vi "Extract IRF (Toeplitz).vi"(4 "balance parameter":dbl=5.0, 6 "Tail Smoothing (T)":bool=TRUE, 7 "Smoothing Order":i32=1, 8 "Error In":errorcluster, 9 "Time Constant":dbl, 10 "Intensity Array":dbl[](array[numeric]), 11 "t Array":dbl[](array[numeric])) -> (0 "Error Out":errorcluster, 1 "Message":string, 2 "IRF Array":dbl[](array[numeric]), 3 "t Array (dup)":dbl[](array[numeric]))   [LabVIEW 2021, in "Fits.lvlib"]
doc: "Extract IRF from provided decay and time constant"
uses:
  Fits.lvlib
  <vilib>/Analysis/baseanly.llb/Matrix Type of Inverse Matrix.ctl
  <vilib>/Analysis/baseanly.llb/A x Vector.vi
  <vilib>/Analysis/7linalg.llb/Create Special Real Matrix.vi
  <vilib>/Analysis/baseanly.llb/Real Inverse Matrix.vi
  <vilib>/Analysis/NI_AALPro.lvlib
  <vilib>/Analysis/NI_AALBase.lvlib
  <vilib>/ErrorRing/Error Ring.xnode
  <vilib>/Utility/error.llb/Error Cluster From Error Code.vi
  Graphs/XY Graph/XY Graph Add-Ons.lvlib
  Math/Math.lvlib
panel:
  out "Tail Min":dbl
  out "Tail Sum":dbl
  out "XY Graph":cluster{"t Array":dbl[], "Array":dbl[]}[](graph)
  # "see the AlliGator License on the block diagram (Ctrl+E or Window:Show Block Diagram)"
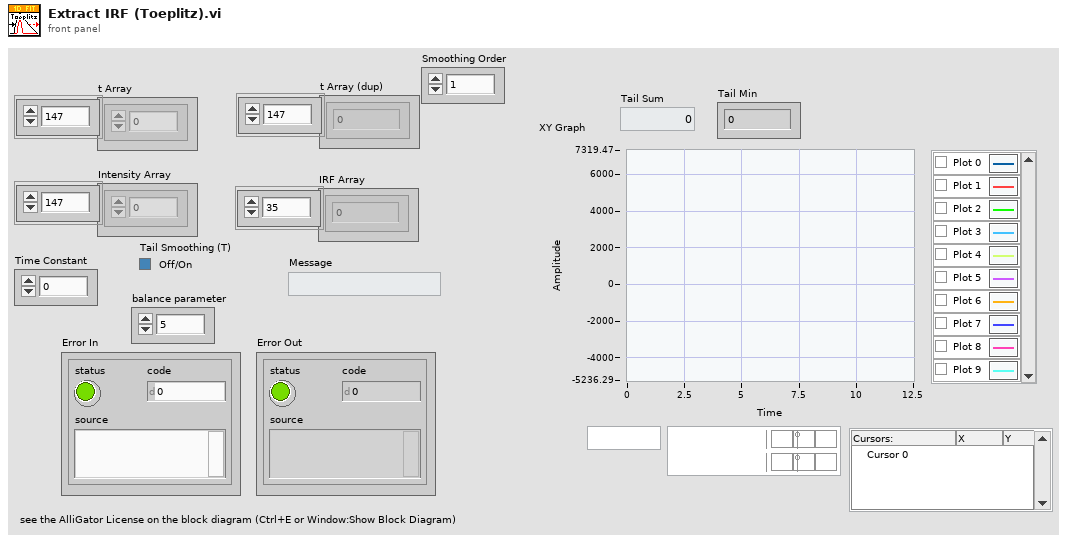
[diagram p1: front panel]
types:
  T1 = typedef "NI_AALBase.lvlib/Matrix Type of Inverse Matrix.ctl" = enum32{"General", "Positive Definite", "Lower Triangular", "Upper Triangular"}
  T2 = enum16{"Positive", "Positive w Noise", "Balanced"}
  T3 = typedef "NI_Matrix.lvlib/RealMatrix.ctl" = dbl[][]
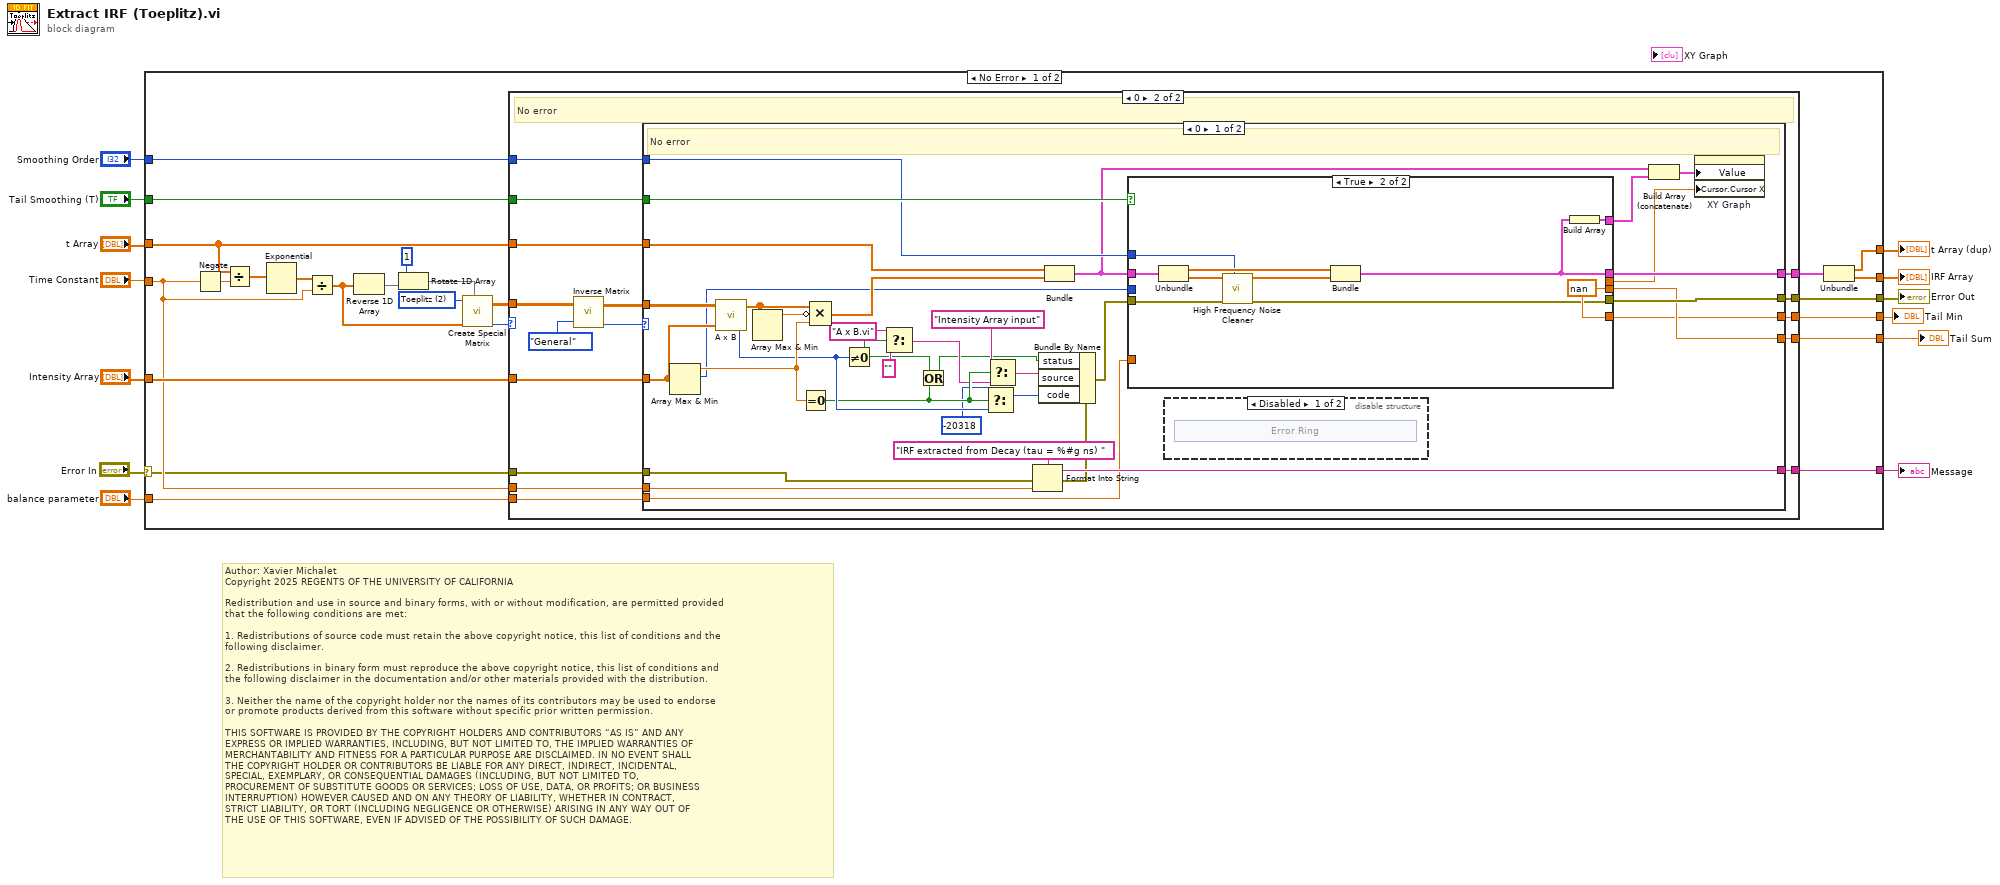
[diagram p0: block diagram]
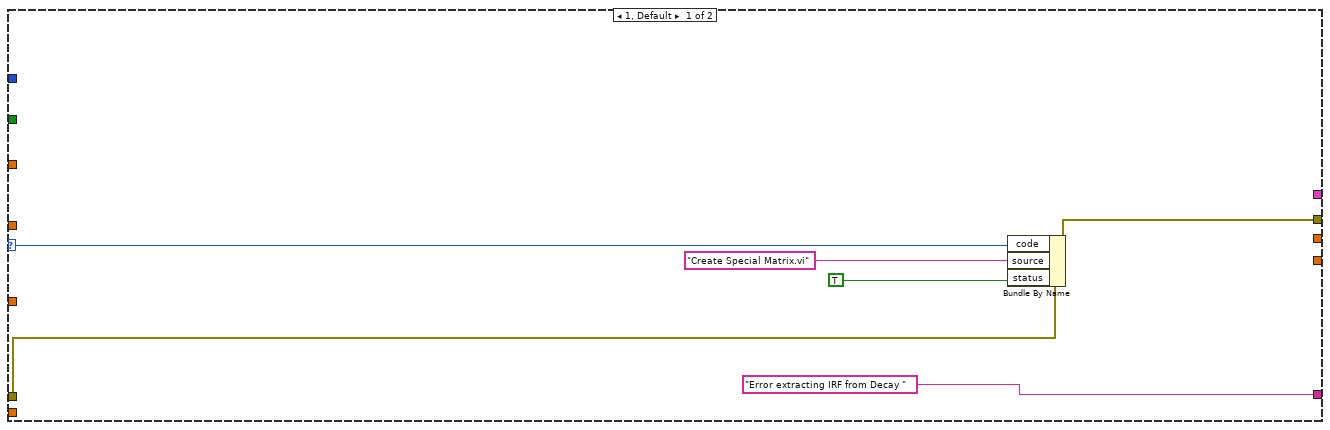
[diagram p2: hidden frame]
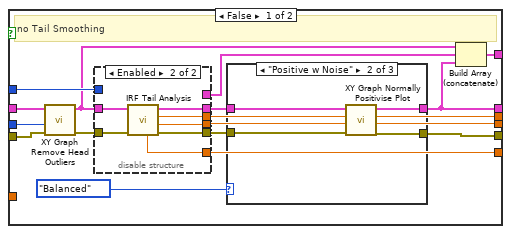
[diagram p4: hidden frame]
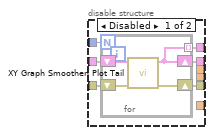
[diagram p5: hidden frame]
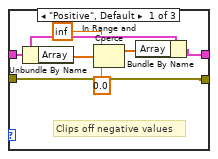
[diagram p6: hidden frame]
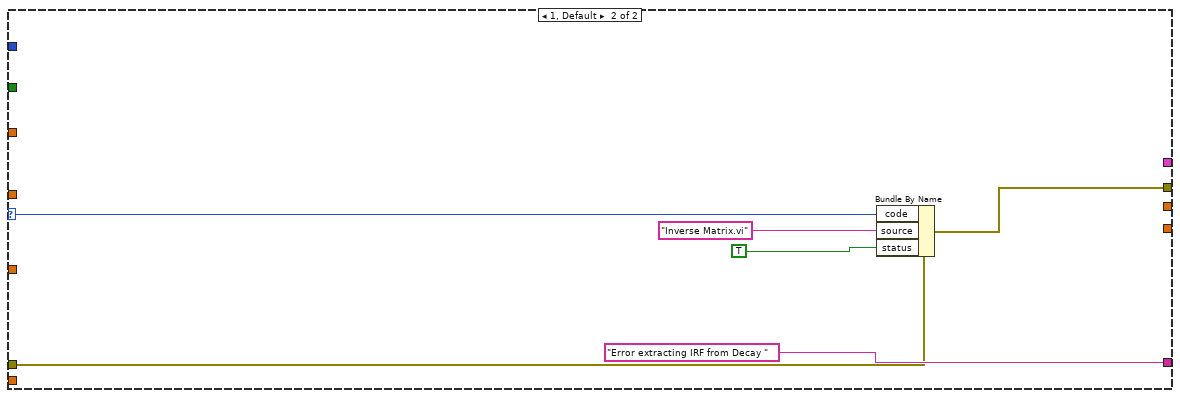
[diagram p8: hidden frame]
diagram:
  # "Author: Xavier Michalet\nCopyright 2025 REGENTS OF THE UNIVERSITY OF CALIFORNIA\n\nRedistribution and use in source and binary forms, with or without modification, are permitted provided\nthat the following conditions are met:\n\n1. Redistributions of source code must retain the above copyright notice, this list of conditions and the\nfollowing disclaimer.\n\n2. Redistributions in binary form must reproduce the above copyright notice, this list of conditions and\nthe following disclaimer in the documentation and/or other materials provided with the distribution.\n\n3. Neither the name of the copyright holder nor the names of its contributors may be used to endorse \nor promote products derived from this software without specific prior written permission.\n\nTHIS SOFTWARE IS PROVIDED BY THE COPYRIGHT HOLDERS AND CONTRIBUTORS “AS IS” AND ANY \nEXPRESS OR IMPLIED WARRANTIES, INCLUDING, BUT NOT LIMITED TO, THE IMPLIED WARRANTIES OF\nMERCHANTABILITY AND FITNESS FOR A PARTICULAR PURPOSE ARE DISCLAIMED. IN NO EVENT SHALL\nTHE COPYRIGHT HOLDER OR CONTRIBUTORS BE LIABLE FOR ANY DIRECT, INDIRECT, INCIDENTAL, \nSPECIAL, EXEMPLARY, OR CONSEQUENTIAL DAMAGES (INCLUDING, BUT NOT LIMITED TO, \nPROCUREMENT OF SUBSTITUTE GOODS OR SERVICES; LOSS OF USE, DATA, OR PROFITS; OR BUSINESS\nINTERRUPTION) HOWEVER CAUSED AND ON ANY THEORY OF LIABILITY, WHETHER IN CONTRACT, \nSTRICT LIABILITY, OR TORT (INCLUDING NEGLIGENCE OR OTHERWISE) ARISING IN ANY WAY OUT OF\nTHE USE OF THIS SOFTWARE, EVEN IF ADVISED OF THE POSSIBILITY OF SUCH DAMAGE."
  n1 = case shown="No Error" "Error In" {
    selector: "Error In" -> [w25 w162]
    tunnel: "Intensity Array" -> [w37 _]
    tunnel: "Time Constant" -> [w29 _]
    tunnel: "t Array" -> [w27 _]
    tunnel: [w24 w162] -> w10
    tunnel: [w30 _] -> w8
    tunnel: "Tail Smoothing (T)" -> [w28 _]
    tunnel: "balance parameter" -> [w26 _]
    tunnel: [w22 _] -> w5
    tunnel: [w21 _] -> w4
    tunnel: "Smoothing Order" -> [w20 _]
    tunnel: [w15 _] -> w2
    tunnel: [w14 _] -> w1
    frame No Error {
      w35 = 2 items=["Identity", "Diagonal", "Toeplitz", "Vandermonde", "Companion", "Hankel", "Hadamard", "Wilkinson", "Hilbert", "Inverse Hilbert", "Rosser", "Pascal"] ("matrix type")
      n2 = Negate(x=w29) -> (-x=w34:dbl)
      n3 = Divide(x=w27, y=w34) -> (x/y=w32:dbl[])
      n4 = Exponential(1:w32) -> (0:w33:dbl[])
      n5 = Divide(x=w33, y=w29) -> (x/y=w19:dbl[])
      n6 = Reverse 1D Array(array=w19) -> (reversed array=w18:dbl[])
      n7 = Rotate 1D Array(1:w18, 2:1 ("n")) -> (0:w17:dbl[])
      n8 = call-poly <vilib>:"Create Special Matrix.vi"("matrix type"=w35, "Input Vector1"=w19, "Input Vector2"=w17) -> ("Special Matrix"=w36:T3, "error"=w31:i32)  [unwired: 2 in]
      n9 = case shown="0" w31 {
        selector: w31 -> [w42 _]
        tunnel: w37 -> [_ w59]
        tunnel: w36 -> [_ w57]
        tunnel: ["Error extracting IRF from Decay " ("Message") w54] -> w30
        tunnel: w29 -> [_ w53]
        tunnel: w28 -> [_ w52]
        tunnel: w27 -> [_ w51]
        tunnel: w26 -> [_ w50]
        tunnel: w25 -> [w40 w49]
        tunnel: [w38 w48] -> w24
        tunnel: [_ w47] -> w23
        tunnel: w20 -> [_ w46]
        tunnel: [_ w45] -> w15
        tunnel: [_ w44] -> w14
        frame 1, Default {
          n10 = Bundle By Name(cluster=w40, "code"=w42, "source"="Create Special Matrix.vi", "status"=TRUE) -> (w38:errorcluster)
        }
        frame 0 {
          # "No error"
          n11 = call-poly <vilib>:"Inverse Matrix.vi"("matrix type"=Matrix_Type_of_Inverse_Matrix."General", "Input Matrix"=w57) -> ("error"=w55:i32, "Inverse Matrix"=w58:T3)
          n12 = case shown="0" w55 {
            selector: w55 -> [_ w160]
            tunnel: w59 -> [w79 _]
            tunnel: w58 -> [w95 _]
            tunnel: [w84 "Error extracting IRF from Decay " ("Message")] -> w54
            tunnel: w53 -> [w82 _]
            tunnel: w52 -> [w81 _]
            tunnel: w51 -> [w78 _]
            tunnel: w50 -> [w77 _]
            tunnel: w49 -> [w68 w157]
            tunnel: [w72 w156] -> w48
            tunnel: [w71 _] -> w47
            tunnel: w46 -> [w70 _]
            tunnel: [w61 _] -> w45
            tunnel: [w60 _] -> w44
            frame 0 {
              # "No error"
              n13 = Array Max & Min(array=w79) -> (max value=w90:dbl, max index (indices)=w67:i32)  [unwired: 2 out]
              n14 = call-poly <vilib>:"A x B.vi"("Vector"=w79, "A"=w95) -> ("error"=w89:i32, "A x Vector"=w92:dbl[])
              n15 = Array Max & Min(array=w92) -> (max value=w91:dbl)  [unwired: 3 out]
              n16 = Equal To 0?(x=w90) -> (x = 0?=w88:bool)
              n17 = Compound Arithmetic op=MULTIPLY(w92, invert w91, w90) -> (w80:dbl[])
              n18 = Not Equal To 0?(x=w89) -> (x != 0?=w85:bool)
              n19 = Select(t="A x B.vi", s=w85, f="") -> (s? t:f=w87:string)
              n20 = Or(x=w85, y=w88) -> (x .or. y?=w74:bool)
              n21 = Select(t=-20318 ("code"), s=w88, f=w89) -> (s? t:f=w75:i32)
              n22 = Select(t="Intensity Array input", s=w88, f=w87) -> (s? t:f=w76:string)
              n23 = Format Into String(format string="IRF extracted from Decay (tau = %#g ns) " ("Message"), error in=w68, w82) -> (resulting string=w84:string, error out=w69:errorcluster)  [unwired: 1 in]
              n24 = Bundle By Name(cluster=w69, "status"=w74, "source"=w76, "code"=w75) -> (w73:errorcluster)
              n25 = Bundle("t Array"=w78, w80) -> (w65:cluster{"t Array":dbl[], dbl[]})  [unwired: 1 in]
              n26 = case shown="True" w81 {
                tunnel: w67 -> [w111 _]
                tunnel: w65 -> [w115 w154]
                tunnel: w77 -> [_ _]
                tunnel: [w104 w148] -> w71
                tunnel: w73 -> [w109 w152]
                tunnel: [w108 w151] -> w72
                tunnel: w70 -> [w112 w146]
                tunnel: [w106 w147] -> w64
                tunnel: [w103 w155] -> w61
                tunnel: [w102 _] -> w62
                tunnel: [w101 w155] -> w60
                frame False {
                  # "no Tail Smoothing"
                  n27 = call "XY Graph Remove Head Outliers.vi"("Error In"=w109, "Peak Index (-1: unknown)"=w111, "Plot in"=w115) -> ("Error Out"=w110:errorcluster, "Plot out"=w107:cluster{"t Array":dbl[], "Array":dbl[]})  [unwired: 6 in, 1 out]
                  n28 = disable-structure shown="Enabled" {
                    disable-tunnel: [w121 w130] -> w114
                    disable-tunnel: [w120 w129] -> w113
                    disable-tunnel: w112 -> [w119 _]
                    disable-tunnel: w110 -> [w118 w131]
                    disable-tunnel: w107 -> [w117 w132]
                    disable-tunnel: [w116 _] -> w105
                    disable-tunnel: [_ w128] -> w103
                    disable-tunnel: [_ w127] -> w102
                    disable-tunnel: [_ w126] -> w101
                    frame Disabled {
                      n29 = for {
                        N: w119 -> [_]
                        shift-right: [w122] -> w121
                        shift-left: w117 -> [w125]
                        shift-right: [w123] -> w120
                        shift-left: w118 -> [w124]
                        tunnel: [w122] -> w116 mode=indexing
                        n30 = call "XY Graph Smoothen Plot Tail.vi"("error in (no error)"=w124, "Plot in"=w125) -> ("error out"=w123:errorcluster, "Plot out"=w122:cluster{"t Array":dbl[], "Y Array":dbl[]})  [unwired: 8 in]
                      }
                    }
                    frame Enabled {
                      n31 = call "IRF Tail Analysis.vi"("error in (no error)"=w131, "Plot in"=w132) -> ("error out"=w129:errorcluster, "Tail Sum"=w128:dbl, "Tail Start"=w127:dbl, "Plot out"=w130:cluster{"t Array":dbl[], "Array":dbl[]}, "Tail Min"=w126:dbl)  [unwired: 5 in]
                    }
                  }
                  n32 = case shown="\"Positive w Noise\"" T2."Balanced" {
                    tunnel: w114 -> [w137 w143 w145]
                    tunnel: w113 -> [w134 w142 w144]
                    tunnel: [w135 w141 w145] -> w104
                    tunnel: [w134 w140 w144] -> w108
                    frame "Positive", Default {
                      # "Clips off negative values"
                      n33 = Unbundle By Name(w137) -> ("Array"=w139:dbl[])
                      n34 = In Range and Coerce(upper limit=inf ("lower limit"), x=w139, lower limit=0.0) -> (coerced(x)=w136:dbl[])  [unwired: 1 out]
                      n35 = Bundle By Name(cluster=w137, "Array"=w136) -> (w135:cluster{"t Array":dbl[], "Array":dbl[]})
                    }
                    frame "Positive w Noise" {
                      n36 = call "XY Graph Normally Positivise Plot.vi"("error in (no error)"=w142, "Plot in"=w143) -> ("error out"=w140:errorcluster, "Plot out"=w141:cluster{"t Array":dbl[], "Array":dbl[]})  [unwired: 8 in]
                    }
                    frame "Balanced" {
                    }
                  }
                  n37 = Build Array (concatenate)(w107, w105, w104) -> (w106:cluster{"t Array":dbl[], "Array":dbl[]}[])
                }
                frame True {
                  w155 = nan ("Tail Sum")
                  n38 = Unbundle(w154) -> ("t Array"=w149:dbl[], w153:dbl[])
                  n39 = call "High Frequency Noise Cleaner.vi"("Repeats"=w146, "Error In"=w152, "Array in"=w153) -> ("Error Out"=w151:errorcluster, "Array out"=w150:dbl[])  [unwired: 7 in]
                  n40 = Bundle("t Array"=w149, "Array out"=w150) -> (w148:cluster{"t Array":dbl[], "Array out":dbl[]})  [unwired: 1 in]
                  n41 = Build Array(w148) -> (w147:cluster{"t Array":dbl[], "Array out":dbl[]}[])
                }
              }
              n42 = disable-structure shown="Disabled" {
                frame Disabled {
                  n43 = xnode "Error Ring"() -> ()  [unwired: 1 out]
                }
                frame Enabled {
                }
              }
              n44 = Build Array (concatenate)(w65, w64) -> (w63:cluster{"t Array":dbl[], "Array out":dbl[]}[])
              n45 = property on="XY Graph" class="XYGraph (strict)"("Value"=w63, "Cursor.Cursor X"=w62) -> ()  [unwired: 2 in, 2 out]
            }
            frame 1, Default {
              n46 = Bundle By Name(cluster=w157, "code"=w160, "source"="Inverse Matrix.vi", "status"=TRUE) -> (w156:errorcluster)
            }
          }
        }
      }
      n47 = Unbundle(w23) -> ("t Array"=w22:dbl[], "Array out"=w21:dbl[])
    }
    frame Error {
    }
  }
  "IRF Array" <- w4
  "Error Out" <- w10
  "t Array (dup)" <- w5
  "Message" <- w8
  "Tail Sum" <- w2
  "Tail Min" <- w1
